vi "Set Speed.vi"(8 "error in (no error)":errorcluster, 10 "Speed (%)":dbl, 11 "Ismatech 3 Channel Settings In":T1={"VISA resource name"="", "Pump Number"=1, "Channel Number"=0, "Simulated?"=TRUE, "Reverse?"=FALSE} {"Channel Number" min=0 max=3; "Pump Number" min=1 max=9}) -> (0 "error out":errorcluster, 1 "Connection Error":bool, 2 "3 Fails":bool, 3 "Ismatech 3 Channel Settings Out":T1={"VISA resource name"="", "Pump Number"=1, "Channel Number"=0, "Simulated?"=TRUE, "Reverse?"=FALSE} {"Channel Number" min=0 max=3; "Pump Number" min=1 max=9})   [LabVIEW 2021, in "Ismatec 4308.lvlib"]
uses:
  Ismatec 4308.lvlib
  Ismatec 4083.ctl
  support/Support Library.lvlib
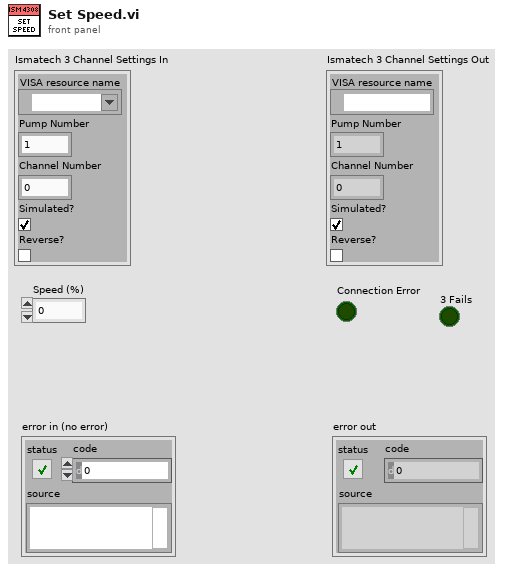
[diagram p1: front panel]
types:
  T1 = typedef "Ismatec 4308.lvlib/Ismatec 4083.ctl" = cluster{"VISA resource name":refnum<visa-resource-name>, "Pump Number":i16, "Channel Number":i16, "Simulated?":bool, "Reverse?":bool}
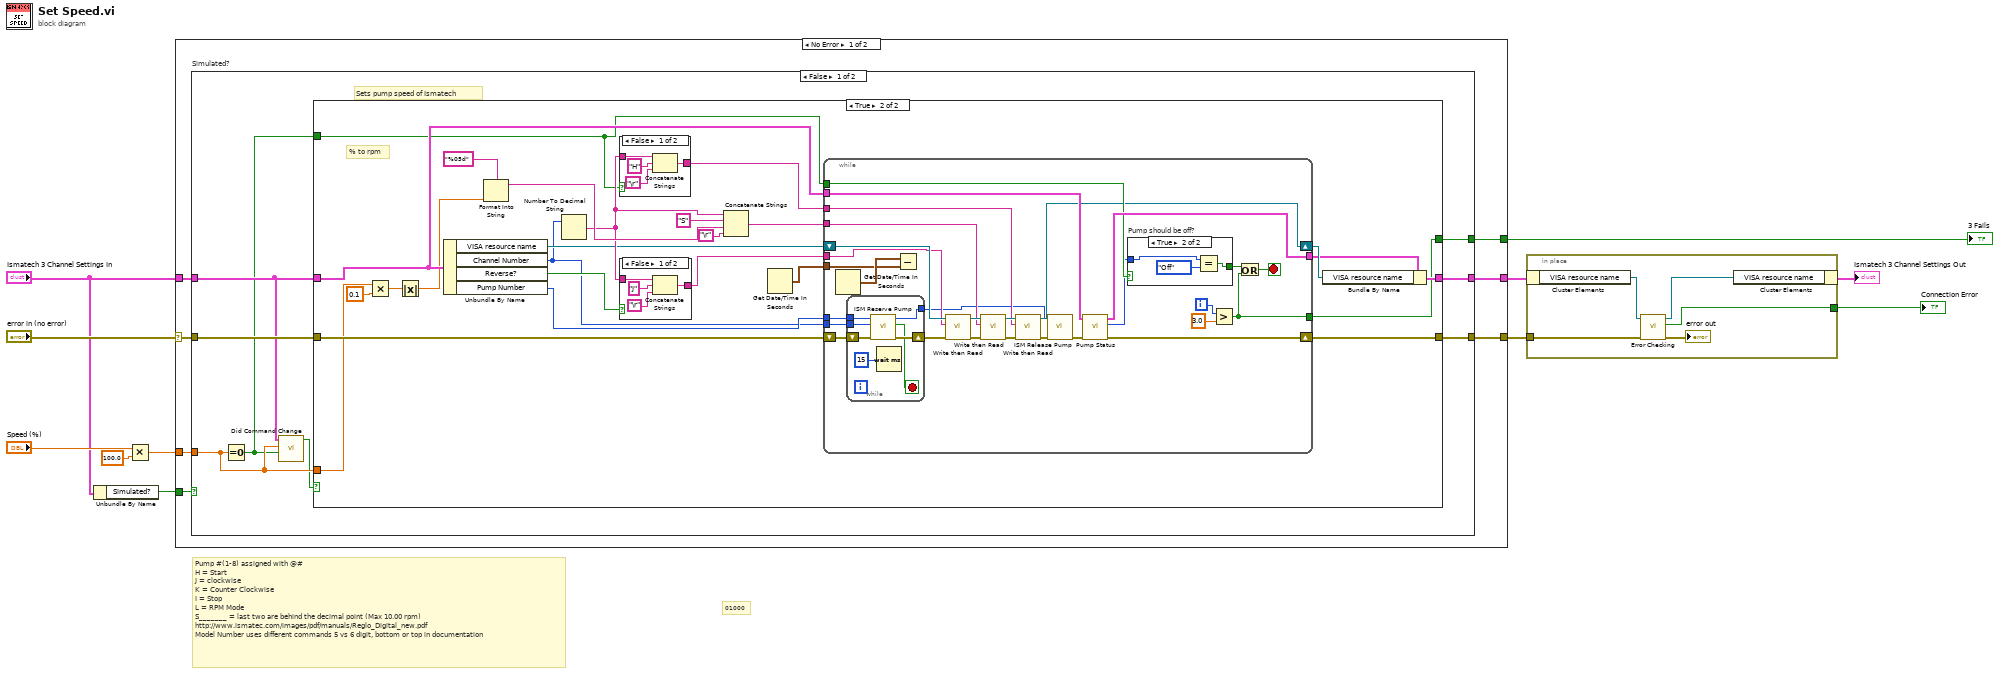
[diagram p0: block diagram]
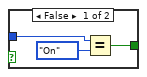
[diagram p3: hidden frame]
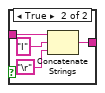
[diagram p4: hidden frame]
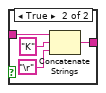
[diagram p5: hidden frame]
diagram:
  # "01000"
  # "Pump #(1-8) assigned with @#\nH = Start\nJ = clockwise\nK = Counter Clockwise\nI = Stop\nL = RPM Mode\nS_______ = last two are behind the decimal point (Max 10.00 rpm)\nhttp://www.ismatec.com/images/pdf/manuals/Reglo_Digital_new.pdf\nModel Number uses different commands 5 vs 6 digit, bottom or top in documentation"
  n1 = Unbundle By Name("Ismatech 3 Channel Settings In") -> ("Simulated?"=w10:bool)
  n2 = Multiply(x="Speed (%)", y=100.0) -> (x*y=w6:dbl)
  n3 = case shown="No Error" "error in (no error)" {
    selector: "error in (no error)" -> [w16 w114]
    tunnel: [w14 w113] -> w4
    tunnel: [w13 w114] -> w9
    tunnel: w6 -> [w15 _]
    tunnel: "Ismatech 3 Channel Settings In" -> [w18 w113]
    tunnel: w10 -> [w17 _]
    tunnel: [w12 _] -> w1
    frame No Error {
      n4 = case "Simulated?" shown="False" w17 {
        tunnel: w15 -> [w22 _]
        tunnel: w18 -> [w23 w112]
        tunnel: [w26 w112] -> w14
        tunnel: w16 -> [w25 w111]
        tunnel: [w24 w111] -> w13
        tunnel: [w19 _] -> w12
        frame False {
          # "Sets pump speed of Ismatech"
          n5 = Equal To 0?(x=w22) -> (x = 0?=w21:bool)
          n6 = call "Did Command Change.vi"("Paused"=w21, "Numeric"=w22, "Ismatech 3 Channel Settings In"=w23) -> ("Change"=w20:bool)  [unwired: 8 in]
          n7 = case shown="True" w20 {
            tunnel: [w28 w53] -> w26
            tunnel: w25 -> [w27 w47]
            tunnel: [w27 w42] -> w24
            tunnel: w22 -> [_ w35]
            tunnel: w23 -> [w28 w34]
            tunnel: w21 -> [_ w32]
            tunnel: [_ w30] -> w19
            frame False {
            }
            frame True {
              # "% to rpm"
              n8 = Multiply(x=w35, y=0.1) -> (x*y=w37:dbl)
              n9 = Absolute Value(x=w37) -> (abs(x)=w33:dbl)
              n10 = Unbundle By Name(w34) -> ("VISA resource name"=w36:refnum<visa-resource-name>, "Channel Number"=w29:i16, "Reverse?"=w43:bool, "Pump Number"=w31:i16)
              n11 = Format Into String(format string="%05d", w33) -> (resulting string=w50:string)  [unwired: 2 in, 1 out]
              n12 = Number To Decimal String(number=w29) -> (decimal integer string=w40:string)  [unwired: 1 in]
              n13 = case shown="False" w32 {
                tunnel: [w96 w99] -> w44
                tunnel: w40 -> [w95 w100]
                frame False {
                  n14 = Concatenate Strings(w95, "H", "\r") -> (w96:string)
                }
                frame True {
                  n15 = Concatenate Strings(w100, "I", "\r") -> (w99:string)
                }
              }
              n16 = case shown="False" w43 {
                tunnel: w40 -> [w105 w110]
                tunnel: [w104 w108] -> w46
                frame False {
                  n17 = Concatenate Strings(w105, "J" ("string"), "\r") -> (w104:string)
                }
                frame True {
                  n18 = Concatenate Strings(w110, "K" ("string"), "\r") -> (w108:string)
                }
              }
              n19 = Concatenate Strings(w40, "S" ("string"), w50, "\r") -> (w45:string)
              n20 = Get Date/Time In Seconds() -> (seconds since 1Jan1904=w38:timestamp)
              n21 = while {
                tunnel: w46 -> [w67]
                tunnel: w45 -> [w65]
                tunnel: w44 -> [w62]
                shift-right: [w81] -> w42
                shift-left: w47 -> [w55]
                shift-right: [w59] -> w41
                shift-left: w36 -> [w68]
                tunnel: w32 -> [w77]
                tunnel: w34 -> [w79]
                tunnel: [w78] -> w39
                tunnel: w38 -> [w72]
                tunnel: w31 -> [w58]
                tunnel: [w71] -> w30
                tunnel: w29 -> [w57]
                i -> [w69]
                stop <- w74 stop-if-true
                n22 = Get Date/Time In Seconds() -> (seconds since 1Jan1904=w73:timestamp)
                n23 = while {
                  tunnel: w58 -> [w86]
                  tunnel: w57 -> [w85]
                  shift-right: [w87] -> w56
                  shift-left: w55 -> [w88]
                  tunnel: [w82] -> w54
                  stop <- w84 stop-if-true
                  n24 = call "ISM Reserve Pump.vi"("error in (no error)"=w88, "ISM Channel # In"=w85, "ISM Pump # In"=w86) -> ("error out"=w87:errorcluster, "Loop Completed"=w84:bool, "ISM Pump # Out"=w82:i32)  [unwired: 6 in]
                  n25 = Wait (ms)(milliseconds to wait=u32 15) -> ()  [unwired: 1 out]
                }
                n26 = Subtract(x=w73, y=w72) -> ()  [unwired: 1 out]
                n27 = call "Write then Read.vi"("error in"=w56, "write buffer"=w67, "VISA resource name in"=w68) -> ("error out"=w64:errorcluster, "VISA resource name out"=w66:refnum<visa-resource-name>)  [unwired: 5 in, 2 out]
                n28 = call "Write then Read.vi"("error in"=w64, "write buffer"=w65, "VISA resource name in"=w66) -> ("error out"=w61:errorcluster, "VISA resource name out"=w63:refnum<visa-resource-name>)  [unwired: 5 in, 2 out]
                n29 = call "Write then Read.vi"("error in"=w61, "write buffer"=w62, "VISA resource name in"=w63) -> ("error out"=w60:errorcluster, "VISA resource name out"=w59:refnum<visa-resource-name>)  [unwired: 5 in, 2 out]
                n30 = call "ISM Release Pump.vi"("error in (no error)"=w60, "Pump Number In"=w54) -> ("error out"=w80:errorcluster)  [unwired: 8 in, 1 out]
                n31 = call "Pump Status.vi"("error in (no error)"=w80, "Ismatech 3 Channel Settings In"=w79) -> ("error out"=w81:errorcluster, "Pump On?"=w70:enum16{"Off", "On", "Not Initialized"}, "Ismatech 3 Channel Settings Out"=w78:T1)  [unwired: 5 in, 2 out]
                n32 = case "Pump should be off?" shown="True" w77 {
                  tunnel: [w89 w92] -> w75
                  tunnel: w70 -> [w90 w93]
                  frame False {
                    n33 = Equal?(x=w90, y=enum16{"Off", "On", "Not Initialized"}."On") -> (x = y?=w89:bool)
                  }
                  frame True {
                    n34 = Equal?(x=w93, y=enum16{"Off", "On", "Not Initialized"}."Off") -> (x = y?=w92:bool)
                  }
                }
                n35 = Greater?(x=w69, y=3.0) -> (0:w71:bool)
                n36 = Or(x=w75, y=w71) -> (x .or. y?=w74:bool)
              }
              n37 = Bundle By Name(cluster=w39, "VISA resource name"=w41) -> (w53:T1)
            }
          }
        }
        frame True {
        }
      }
    }
    frame Error {
    }
  }
  "3 Fails" <- w1
  n38 = in-place {
    in-place-border: w9 -> [w119]
    in-place-border: [w117] -> w5
    n39 = in-place-cluster #1(w4) -> ("VISA resource name"=w116:refnum<visa-resource-name>)
    n40 = call "Error Checking.vi"("error in (no error)"=w119, "VISA resource name"=w116) -> ("error out"=→"error out":errorcluster, "Connection Error"=w117:bool, "VISA resource name"=w115:refnum<visa-resource-name>)  [unwired: 7 in]
    n41 = in-place-cluster #1("VISA resource name"=w115) -> (→"Ismatech 3 Channel Settings Out":T1)
  }
  "Connection Error" <- w5
